vi "Get Item From Index.vi"(8 "error in (no error)":errorcluster caption="错误输入（无错误）", 9 "Index":i32, 11 "具体聚集 输入":refnum<class "具体聚集.lvclass"> caption="DNL_LabVIEW Object in") -> (0 "error out":errorcluster caption="错误输出", 1 "迭代器.lvlib:雇员.lvclass":refnum<class "雇员.lvclass">, 3 "具体聚集 输出":refnum<class "具体聚集.lvclass"> caption="DNL_LabVIEW Object out")   [LabVIEW 2011, in "迭代器.lvlib" / "具体聚集.lvclass"]
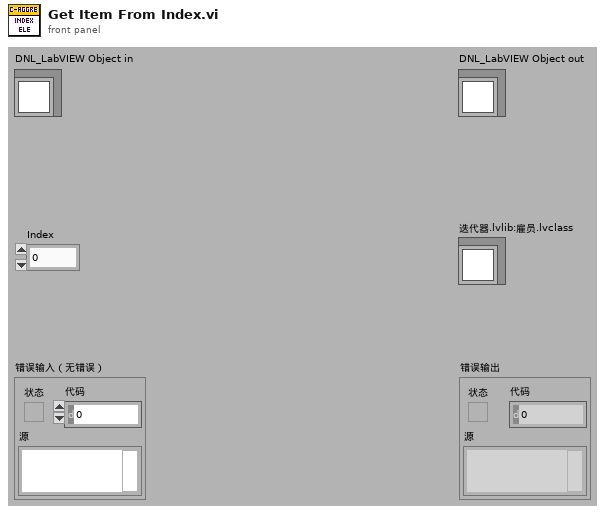
[diagram p1: front panel]
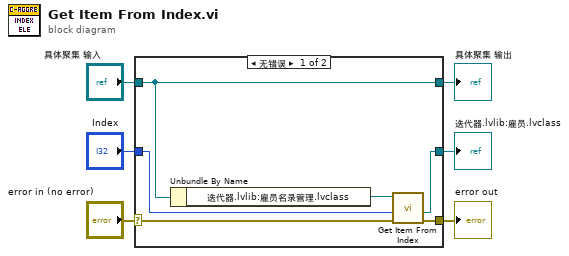
[diagram p0: block diagram]
diagram:
  n1 = case shown="无错误" "error in (no error)" {
    selector: "error in (no error)" -> [w10 w14]
    tunnel: [w8 w14] -> w5
    tunnel: [w12 w13] -> w3
    tunnel: "具体聚集 输入" -> [w12 w13]
    tunnel: "Index" -> [w9 _]
    tunnel: [w7 _] -> w1
    frame No Error {
      n2 = Unbundle By Name(w12) -> ("迭代器.lvlib:雇员名录管理.lvclass"=w11:refnum<class "雇员名录管理.lvclass">)
      n3 = call "Get Item From Index.vi"("error in (no error)"=w10, "数值"=w9, "雇员名录管理 输入"=w11) -> ("error out"=w8:errorcluster, "迭代器.lvlib:雇员.lvclass"=w7:refnum<class "雇员.lvclass">)  [unwired: 6 in, 1 out]
    }
    frame Error {
    }
  }
  "error out" <- w5
  "具体聚集 输出" <- w3
  "迭代器.lvlib:雇员.lvclass" <- w1
